vi "LAbview proje.vi"() -> ()   [LabVIEW 2017]
uses:
  <vilib>/Instr/_visa.llb/VISA Configure Serial Port (Instr).vi
panel:
  out "Hava Kalitesi Grafiği":dbl(graph)
  in  "stop":bool
  out "Bağlantı":errorcluster
  out "Hava Kalitesi":string
  in  "Portu seçiniz.":refnum<visa-resource-name>
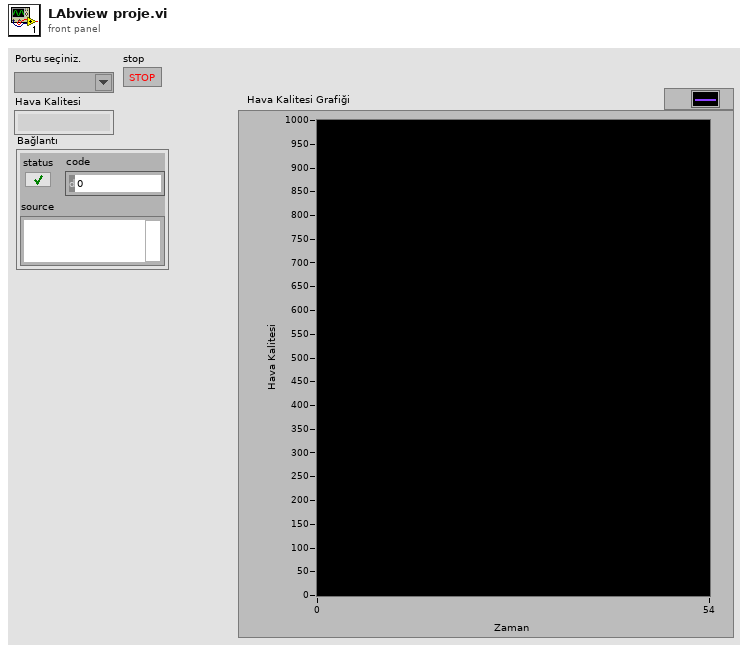
[diagram p1: front panel]
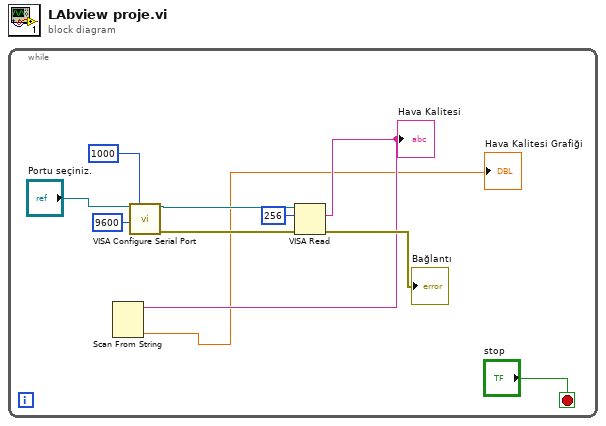
[diagram p0: block diagram]
diagram:
  n1 = while {
    stop <- "stop" stop-if-true
    n2 = call-poly "VISA Configure Serial Port"("VISA resource name"="Portu seçiniz.", "timeout (10sec)"=u32 1000, "baud rate (9600)"=u32 9600) -> ("VISA resource name out"=w6:refnum<visa-resource-name>, "error out"=w5:errorcluster)  [unwired: 11 in]
    n3 = VISA Read(VISA resource name=w6, byte count=u32 256, error in (no error)=w5) -> (read buffer=w2:string, error out=→"Bağlantı":errorcluster)  [unwired: 2 out]
    "Hava Kalitesi" <- w2
    n4 = Scan From String(input string=w2) -> (output 1=→"Hava Kalitesi Grafiği":dbl)  [unwired: 4 in, 3 out]
  }
